vi "Write.vi"(8 "error in (no error)":errorcluster, 9 "timeout ms (25000)":i32, 10 "Data":string, 11 "connection ID":refnum<k5>) -> (0 "error out":errorcluster, 3 "connection ID out":refnum<k5>)   [LabVIEW 2013, in "WebSockets.lvlib"]
doc: "Sends a WebSocket message to the client."
uses:
  WebSockets.lvlib
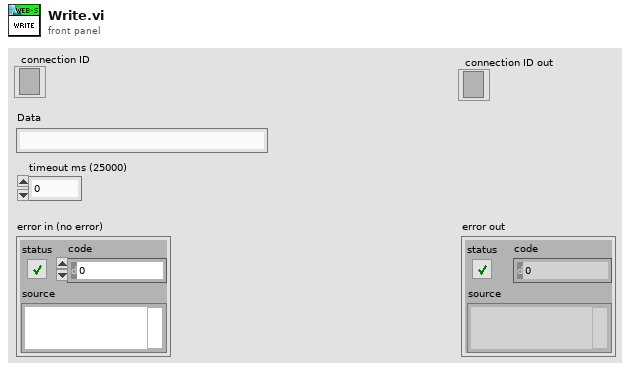
[diagram p1: front panel]
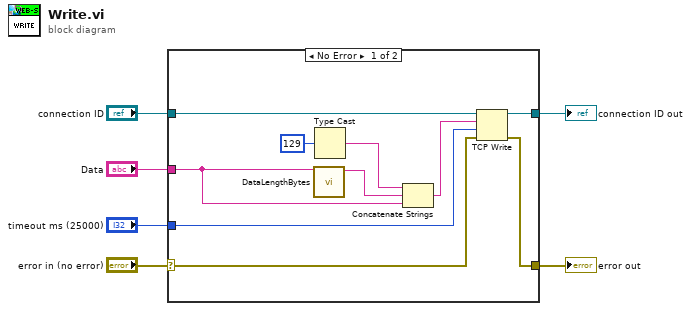
[diagram p0: block diagram]
diagram:
  n1 = case shown="No Error" "error in (no error)" {
    selector: "error in (no error)" -> [w13 w18]
    tunnel: [w14 w18] -> w5
    tunnel: [w16 w17] -> w3
    tunnel: "connection ID" -> [w15 w17]
    tunnel: "Data" -> [w10 _]
    tunnel: "timeout ms (25000)" -> [w7 _]
    frame No Error {
      n2 = call "DataLengthBytes.vi"("Data"=w10) -> ("Length Bytes"=w11:string)  [unwired: 10 in]
      n3 = Type Cast(x=u8 129) -> (*(type *) &x=w9:string)  [unwired: 1 in]
      n4 = Concatenate Strings(w9, w11, w10) -> (w8:string)
      n5 = TCP Write(connection ID=w15, data in=w8, error in (no error)=w13, 9:w7) -> (connection ID out=w16:refnum<k5>, error out=w14:errorcluster)  [unwired: 1 out]
    }
    frame Error {
    }
  }
  "connection ID out" <- w3
  "error out" <- w5
